vi "measurement_data_conversion_factor.vi"() -> (0 "MATLAB function handler":string[](array[string]))   [LabVIEW 2017]
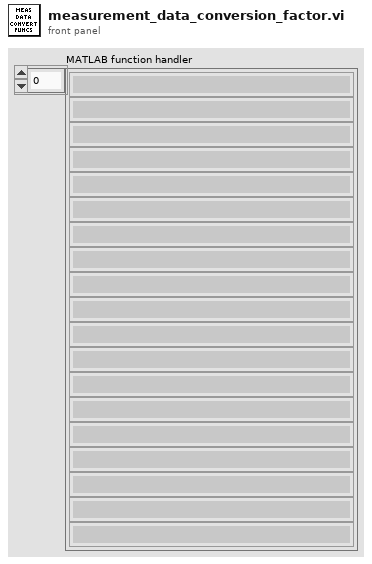
[diagram p1: front panel]
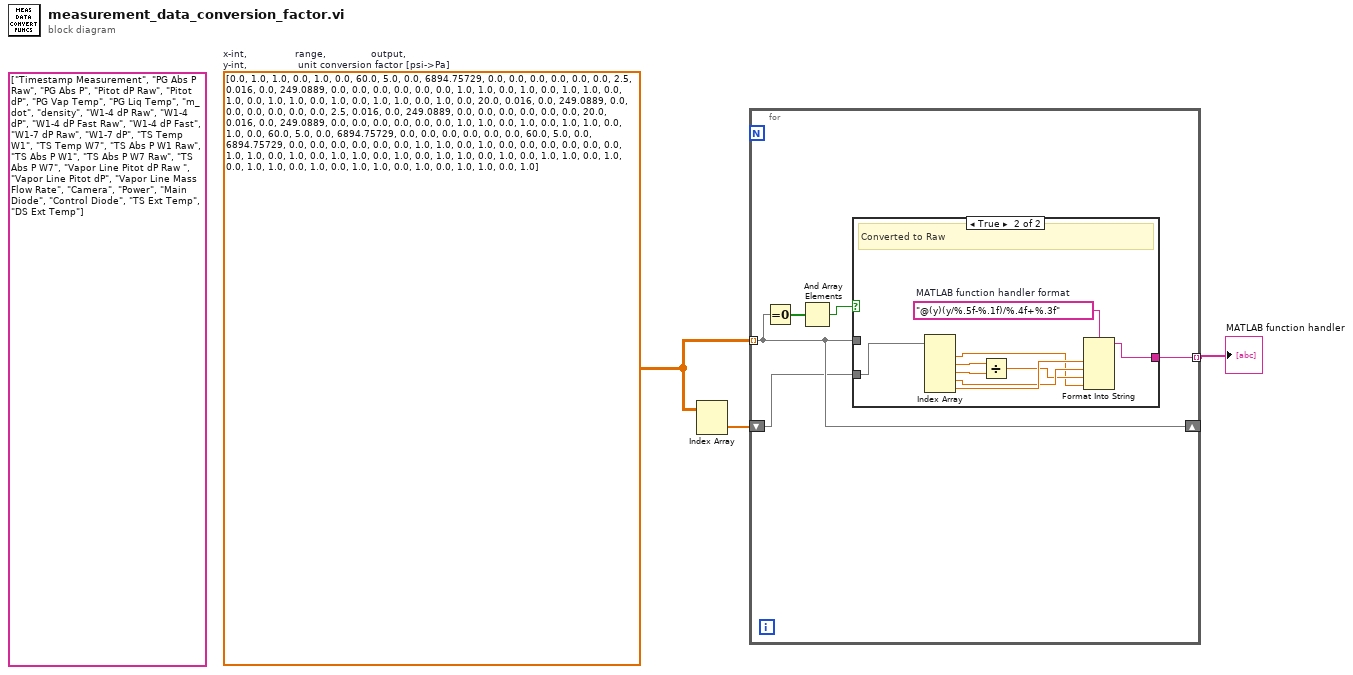
[diagram p0: block diagram]
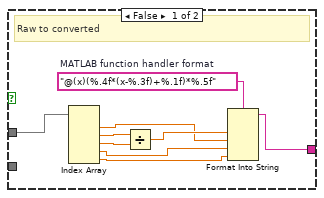
[diagram p2: hidden frame]
diagram:
  w3 = dbl[][] [[0.0, 1.0, 1.0, 0.0, 1.0], [0.0, 60.0, 5.0, 0.0, 6894.75729], [0.0, 0.0, 0.0, 0.0, 0.0], [0.0, 2.5, 0.016, 0.0, 249.0889], [0.0, 0.0, 0.0, 0.0, 0.0], [0.0, 1.0, 1.0, 0.0, 1.0], [0.0, 1.0, 1.0, 0.0, 1.0], [0.0, 1.0, 1.0, 0.0, 1.0], [0.0, 1.0, 1.0, 0.0, 1.0], [0.0, 20.0, 0.016, 0.0, 249.0889], [0.0, 0.0, 0.0, 0.0, 0.0], [0.0, 2.5, 0.016, 0.0, 249.0889], [0.0, 0.0, 0.0, 0.0, 0.0], [0.0, 20.0, 0.016, 0.0, 249.0889], [0.0, 0.0, 0.0, 0.0, 0.0], [0.0, 1.0, 1.0, 0.0, 1.0], [0.0, 1.0, 1.0, 0.0, 1.0], [0.0, 60.0, 5.0, 0.0, 6894.75729], [0.0, 0.0, 0.0, 0.0, 0.0], [0.0, 60.0, 5.0, 0.0, 6894.75729], [0.0, 0.0, 0.0, 0.0, 0.0], [0.0, 1.0, 1.0, 0.0, 1.0], [0.0, 0.0, 0.0, 0.0, 0.0], [0.0, 1.0, 1.0, 0.0, 1.0], [0.0, 1.0, 1.0, 0.0, 1.0], [0.0, 1.0, 1.0, 0.0, 1.0], [0.0, 1.0, 1.0, 0.0, 1.0], [0.0, 1.0, 1.0, 0.0, 1.0], [0.0, 1.0, 1.0, 0.0, 1.0], [0.0, 1.0, 1.0, 0.0, 1.0]]  # x-int,                range,               output,           y-int,                 unit conversion factor [psi->Pa]
  (unwired) string[] ["Timestamp Measurement", "PG Abs P Raw", "PG Abs P", "Pitot dP Raw", "Pitot dP", "PG Vap Temp", "PG Liq Temp", "m_dot", "density", "W1-4 dP Raw", "W1-4 dP", "W1-4 dP Fast Raw", "W1-4 dP Fast", "W1-7 dP Raw", "W1-7 dP", "TS Temp W1", "TS Temp W7", "TS Abs P W1 Raw", "TS Abs P W1", "TS Abs P W7 Raw", "TS Abs P W7", "Vapor Line Pitot dP Raw ", "Vapor Line Pitot dP", "Vapor Line Mass Flow Rate", "Camera", "Power", "Main Diode", "Control Diode", "TS Ext Temp", "DS Ext Temp"]
  n1 = Index Array(array=w3) -> (element=w2:dbl[])  [unwired: 2 in]
  n2 = for {
    tunnel: w3 -> [w7] mode=indexing
    tunnel: [w8] -> w1 mode=indexing
    shift-right: [w7] -> _
    shift-left: w2 -> [w5]
    n3 = Equal To 0?(x=w7) -> (x = 0?=w6:bool[])
    n4 = And Array Elements(Boolean array=w6) -> (logical AND=w4:bool)
    n5 = case shown="True" w4 {
      tunnel: [w10 w18] -> w8
      tunnel: w7 -> [w9 _]
      tunnel: w5 -> [_ w19]
      frame False {
        w13 = "@(x)(%.4f*(x-%.3f)+%.1f)*%.5f"  # MATLAB function handler format
        # "Raw to converted"
        n6 = Index Array(array=w9) -> (element #1=w11:dbl, element #2=w17:dbl, element #3=w16:dbl, element #4=w15:dbl, element #5=w14:dbl)  [unwired: 5 in]
        n7 = Divide(x=w17, y=w16) -> (x/y=w12:dbl)
        n8 = Format Into String(format string=w13, w12, w11, w15, w14) -> (resulting string=w10:string)  [unwired: 2 in, 1 out]
      }
      frame True {
        w24 = "@(y)(y/%.5f-%.1f)/%.4f+%.3f"  # MATLAB function handler format
        # "Converted to Raw"
        n9 = Index Array(array=w19) -> (element #1=w20:dbl, element #2=w26:dbl, element #3=w25:dbl, element #4=w22:dbl, element #5=w23:dbl)  [unwired: 5 in]
        n10 = Divide(x=w26, y=w25) -> (x/y=w21:dbl)
        n11 = Format Into String(format string=w24, w23, w22, w21, w20) -> (resulting string=w18:string)  [unwired: 2 in, 1 out]
      }
    }
  }
  "MATLAB function handler" <- w1
